vi "Test Get Specific Symbol.vi"(8 "error in (no error)":errorcluster, 11 "Test Case In":refnum<class "Conditional Disabled Configurator Test.lvclass">) -> (0 "error out":errorcluster, 3 "Test Case Out":refnum<class "Conditional Disabled Configurator Test.lvclass">)   [LabVIEW 2020, in "Conditional Disabled Configurator Test.lvclass"]
uses:
  Conditional Disabled Configurator Test.lvclass
  Conditional Disabled Configurator Test.lvclass/Conditional Disabled Configurator Test.ctl
  01074fa8-ee8a-411d-bc8b-fc92c4f90959.vi
  source/Conditional Disabled Configurator/Conditional Disabled Configurator.lvclass
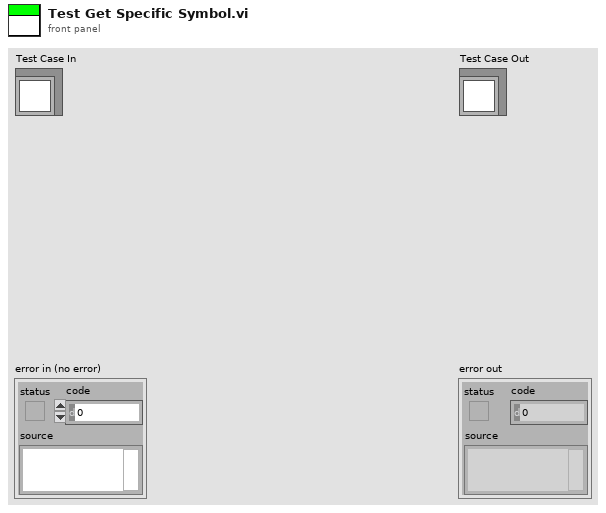
[diagram p1: front panel]
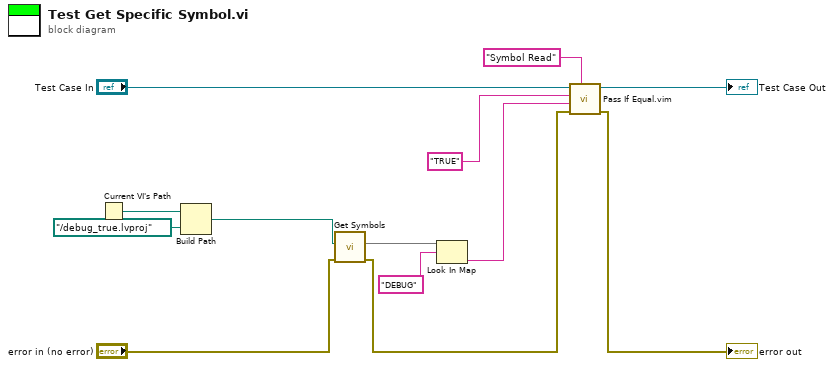
[diagram p0: block diagram]
diagram:
  n1 = Current VI's Path() -> (path=w10:path)
  n2 = Build Path(base path=w10, name or relative path=path "../debug_true.lvproj") -> (appended path=w8:path)
  n3 = call "Get Symbols.vi"("error in (no error)"="error in (no error)", "Project Path"=w8) -> ("error out"=w6:errorcluster, "Symbols"=w5:map{string, string})  [unwired: 8 in]
  n4 = Look In Map(map=w5, key="DEBUG") -> (value=w3:string)  [unwired: 1 in, 1 out]
  n5 = call "Pass If Equal.vim"("Description"="Symbol Read", "error in (no error)"=w6, "Actual"=w3, "Expected"="TRUE", "LUnit Test Case In"="Test Case In") -> ("error out"=→"error out":errorcluster, "LUnit Test Case Out"=→"Test Case Out":refnum<class "Conditional Disabled Configurator Test.lvclass">)  [unwired: 5 in]
